vi "GeoData.vi"() -> ()   [LabVIEW 2017] (continued)
KS\tCloud County\tH1\n67466\t20029\tMiltonvale\tKS\tCloud County\tH1\n67417\t20029\tAurora\tKS\tCloud County\tH1\n66930\t20029\tAgenda\tKS\tCloud County\tH1\n67420\t20029\tBeloit\tKS\tCloud County\tH1\n66948\t20029\tJamestown\tKS\tCloud County\tH1\n67436\t20029\tDelphos\tKS\tCloud County\tH1\n67445\t20029\tGlasco\tKS\tCloud County\tH1\n66938\t20029\tClyde\tKS\tCloud County\tH1\n66783\t20031\tYates center\tKS\tCoffey County\tH1\n66868\t20031\tReading\tKS\tCoffey County\tH1\n66093\t20031\tWestphalia\tKS\tCoffey County\tH1\n66854\t20031\tHartford\tKS\tCoffey County\tH1\n66856\t20031\tLebo\tKS\tCoffey County\tH1\n66839\t20031\tBurlington\tKS\tCoffey County\tH1\n66864\t20031\tNeosho rapids\tKS\tCoffey County\tH1\n66857\t20031\tLe roy\tKS\tCoffey County\tH1\n66095\t20031\tWilliamsburg\tKS\tCoffey County\tH1\n66852\t20031\tGridley\tKS\tCoffey County\tH1\n66758\t20031\tNeosho falls\tKS\tCoffey County\tH1\n66871\t20031\tWaverly\tKS\tCoffey County\tH1\n67029\t20033\tColdwater\tKS\tComanche County\tH1\n67155\t20033\tWilmore\tKS\tComanche County\tH1\n67127\t20033\tProtection\tKS\tComanche County\tH1\n67005\t20035\tArkansas city\tKS\tCowley County\tH1\n67119\t20035\tOxford\tKS\tCowley County\tH1\n67110\t20035\tMulvane\tKS\tCowley County\tH1\n67072\t20035\tLatham\tKS\tCowley County\tH1\n67102\t20035\tMaple city\tKS\tCowley County\tH1\n67008\t20035\tAtlanta\tKS\tCowley County\tH1\n67051\t20035\tGeuda springs\tKS\tCowley County\tH1\n67023\t20035\tCambridge\tKS\tCowley County\tH1\n67039\t20035\tDouglass\tKS\tCowley County\tH1\n67024\t20035\tCedar vale\tKS\tCowley County\tH1\n67131\t20035\tRock\tKS\tCowley County\tH1\n67038\t20035\tDexter\tKS\tCowley County\tH1\n67146\t20035\tUdall\tKS\tCowley County\tH1\n67156\t20035\tWinfield\tKS\tCowley County\tH1\n67019\t20035\tBurden\tKS\tCowley County\tH1\n66712\t20037\tArma\tKS\tCrawford County\tH1\n66746\t20037\tHepler\tKS\tCrawford County\tH1\n66701\t20037\tFort scott\tKS\tCrawford County\tH1\n66743\t20037\tGirard\tKS\tCrawford County\tH1\n66711\t20037\tArcadia\tKS\tCrawford County\tH1\n66724\t20037\tCherokee\tKS\tCrawford County\tH1\n66734\t20037\tFarlington\tKS\tCrawford County\tH1\n66760\t20037\tOpolis\tKS\tCrawford County\tH1\n66763\t20037\tFrontenac\tKS\tCrawford County\tH1\n66756\t20037\tMulberry\tKS\tCrawford County\tH1\n66762\t20037\tPittsburg\tKS\tCrawford County\tH1\n66735\t20037\tFranklin\tKS\tCrawford County\tH1\n66781\t20037\tWeir\tKS\tCrawford County\tH1\n66753\t20037\tMc cune\tKS\tCrawford County\tH1\n66780\t20037\tWalnut\tKS\tCrawford County\tH1\n67749\t20039\tOberlin\tKS\tDecatur County\tH1\n67757\t20039\tSelden\tKS\tDecatur County\tH1\n67643\t20039\tJennings\tKS\tDecatur County\tH1\n67653\t20039\tNorcatur\tKS\tDecatur County\tH1\n67635\t20039\tDresden\tKS\tDecatur County\tH1\n66441\t20041\tJunction city\tKS\tDickinson County\tH1\n67410\t20041\tAbilene\tKS\tDickinson County\tH1\n67448\t20041\tGypsum\tKS\tDickinson County\tH1\n67451\t20041\tHope\tKS\tDickinson County\tH1\n67480\t20041\tSolomon\tKS\tDickinson County\tH1\n67475\t20041\tRamona\tKS\tDickinson County\tH1\n67449\t20041\tHerington\tKS\tDickinson County\tH1\n67441\t20041\tEnterprise\tKS\tDickinson County\tH1\n67492\t20041\tWoodbine\tKS\tDickinson County\tH1\n67431\t20041\tChapman\tKS\tDickinson County\tH1\n67487\t20041\tWakefield\tKS\tDickinson County\tH1\n67482\t20041\tTalmage\tKS\tDickinson County\tH1\n66094\t20043\tWhite cloud\tKS\tDoniphan County\tH1\n66087\t20043\tTroy\tKS\tDoniphan County\tH1\n66017\t20043\tDenton\tKS\tDoniphan County\tH1\n66090\t20043\tWathena\tKS\tDoniphan County\tH1\n66024\t20043\tElwood\tKS\tDoniphan County\tH1\n66041\t20043\tLancaster\tKS\tDoniphan County\tH1\n66008\t20043\tBendena\tKS\tDoniphan County\tH1\n66035\t20043\tHighland\tKS\tDoniphan County\tH1\n66002\t20043\tAtchison\tKS\tDoniphan County\tH1\n66532\t20043\tRobinson\tKS\tDoniphan County\tH1\n66049\t20045\tLawrence\tKS\tDouglas County\tH1\n66025\t20045\tEudora\tKS\tDouglas County\tH1\n66050\t20045\tLecompton\tKS\tDouglas County\tH1\n66046\t20045\tLawrence\tKS\tDouglas County\tH1\n66092\t20045\tWellsville\tKS\tDouglas County\tH1\n66021\t20045\tEdgerton\tKS\tDouglas County\tH1\n66409\t20045\tBerryton\tKS\tDouglas County\tH1\n66524\t20045\tOverbrook\tKS\tDouglas County\tH1\n66047\t20045\tLawrence\tKS\tDouglas County\tH1\n66542\t20045\tTecumseh\tKS\tDouglas County\tH1\n66045\t20045\tLawrence\tKS\tDouglas County\tH1\n66006\t20045\tBaldwin city\tKS\tDouglas County\tH1\n66044\t20045\tLawrence\tKS\tDouglas County\tH1\n67054\t20047\tGreensburg\tKS\tEdwards County\tH1\n67563\t20047\tOfferle\tKS\tEdwards County\tH1\n67519\t20047\tBelpre\tKS\tEdwards County\tH1\n67059\t20047\tHaviland\tKS\tEdwards County\tH1\n67547\t20047\tKinsley\tKS\tEdwards County\tH1\n67557\t20047\tMacksville\tKS\tEdwards County\tH1\n67552\t20047\tLewis\tKS\tEdwards County\tH1\n67344\t20049\tElk city\tKS\tElk County\tH1\n67353\t20049\tMoline\tKS\tElk County\tH1\n67345\t20049\tElk falls\tKS\tElk County\tH1\n67346\t20049\tGrenola\tKS\tElk County\tH1\n67122\t20049\tPiedmont\tKS\tElk County\tH1\n67137\t20049\tSevery\tKS\tElk County\tH1\n67047\t20049\tFall river\tKS\tElk County\tH1\n67349\t20049\tHoward\tKS\tElk County\tH1\n67352\t20049\tLongton\tKS\tElk County\tH1\n67640\t20051\tGorham\tKS\tEllis County\tH1\n67659\t20051\tPenokee\tKS\tEllis County\tH1\n67660\t20051\tPfeifer\tKS\tEllis County\tH1\n67651\t20051\tNatoma\tKS\tEllis County\tH1\n67663\t20051\tPlainville\tKS\tEllis County\tH1\n67627\t20051\tCatharine\tKS\tEllis County\tH1\n67671\t20051\tVictoria\tKS\tEllis County\tH1\n67667\t20051\tSchoenchen\tKS\tEllis County\tH1\n67601\t20051\tHays\tKS\tEllis County\tH1\n67674\t20051\tWalker\tKS\tEllis County\tH1\n67637\t20051\tEllis\tKS\tEllis County\tH1\n67556\t20051\tMc cracken\tKS\tEllis County\tH1\n67520\t20051\tBison\tKS\tEllis County\tH1\n67423\t20053\tBeverly\tKS\tEllsworth County\tH1\n67459\t20053\tLorraine\tKS\tEllsworth County\tH1\n67450\t20053\tHolyrood\tKS\tEllsworth County\tH1\n67439\t20053\tEllsworth\tKS\tEllsworth County\tH1\n67425\t20053\tBrookville\tKS\tEllsworth County\tH1\n67444\t20053\tGeneseo\tKS\tEllsworth County\tH1\n67490\t20053\tWilson\tKS\tEllsworth County\tH1\n67427\t20053\tBushton\tKS\tEllsworth County\tH1\n67464\t20053\tMarquette\tKS\tEllsworth County\tH1\n67454\t20053\tKanopolis\tKS\tEllsworth County\tH1\n67851\t20055\tHolcomb\tKS\tFinney County\tH1\n67839\t20055\tDighton\tKS\tFinney County\tH1\n67838\t20055\tDeerfield\tKS\tFinney County\tH1\n67871\t20055\tScott city\tKS\tFinney County\tH1\n67853\t20055\tIngalls\tKS\tFinney County\tH1\n67868\t20055\tPierceville\tKS\tFinney County\tH1\n67846\t20055\tGarden city\tKS\tFinney County\tH1\n67835\t20055\tCimarron\tKS\tFinney County\tH1\n67834\t20057\tBucklin\tKS\tFord County\tH1\n67563\t20057\tOfferle\tKS\tFord County\tH1\n67842\t20057\tFord\tKS\tFord County\tH1\n67844\t20057\tFowler\tKS\tFord County\tH1\n67865\t20057\tMinneola\tKS\tFord County\tH1\n67801\t20057\tDodge city\tKS\tFord County\tH1\n67882\t20057\tWright\tKS\tFord County\tH1\n67876\t20057\tSpearville\tKS\tFord County\tH1\n67841\t20057\tEnsign\tKS\tFord County\tH1\n67835\t20057\tCimarron\tKS\tFord County\tH1\n66033\t20059\tGreeley\tKS\tFranklin County\tH1\n66079\t20059\tRantoul\tKS\tFranklin County\tH1\n66076\t20059\tPomona\tKS\tFranklin County\tH1\n66078\t20059\tPrinceton\tKS\tFranklin County\tH1\n66092\t20059\tWellsville\tKS\tFranklin County\tH1\n66080\t20059\tRichmond\tKS\tFranklin County\tH1\n66524\t20059\tOverbrook\tKS\tFranklin County\tH1\n66067\t20059\tOttawa\tKS\tFranklin County\tH1\n66095\t20059\tWilliamsburg\tKS\tFranklin County\tH1\n66042\t20059\tLane\tKS\tFranklin County\tH1\n66528\t20059\tQuenemo\tKS\tFranklin County\tH1\n66006\t20059\tBaldwin city\tKS\tFranklin County\tH1\n66064\t20059\tOsawatomie\tKS\tFranklin County\tH1\n66441\t20061\tJunction city\tKS\tGeary County\tH1\n66442\t20061\tFort riley\tKS\tGeary County\tH1\n66401\t20061\tAlma\tKS\tGeary County\tH1\n66834\t20061\tAlta vista\tKS\tGeary County\tH1\n66502\t20061\tManhattan\tKS\tGeary County\tH1\n66849\t20061\tDwight\tKS\tGeary County\tH1\n66872\t20061\tWhite city\tKS\tGeary County\tH1\n67431\t20061\tChapman\tKS\tGeary County\tH1\n66514\t20061\tMilford\tKS\tGeary County\tH1\n67487\t20061\tWakefield\tKS\tGeary County\tH1\n67748\t20063\tOakley\tKS\tGove County\tH1\n67752\t20063\tQuinter\tKS\tGove County\tH1\n67751\t20063\tPark\tKS\tGove County\tH1\n67738\t20063\tGrinnell\tKS\tGove County\tH1\n67737\t20063\tGrainfield\tKS\tGove County\tH1\n67736\t20063\tGove\tKS\tGove County\tH1\n67625\t20065\tBogue\tKS\tGraham County\tH1\n67656\t20065\tOgallah\tKS\tGraham County\tH1\n67650\t20065\tMorland\tKS\tGraham County\tH1\n67659\t20065\tPenokee\tKS\tGraham County\tH1\n67642\t20065\tHill city\tKS\tGraham County\tH1\n67740\t20065\tHoxie\tKS\tGraham County\tH1\n67632\t20065\tDamar\tKS\tGraham County\tH1\n67657\t20065\tPalco\tKS\tGraham County\tH1\n67672\t20065\tWakeeney\tKS\tGraham County\tH1\n67855\t20067\tJohnson\tKS\tGrant County\tH1\n67880\t20067\tUlysses\tKS\tGrant County\tH1\n67870\t20067\tSatanta\tKS\tGrant County\tH1\n67860\t20067\tLakin\tKS\tGrant County\tH1\n67844\t20069\tFowler\tKS\tGray County\tH1\n67853\t20069\tIngalls\tKS\tGray County\tH1\n67801\t20069\tDodge city\tKS\tGray County\tH1\n67867\t20069\tMontezuma\tKS\tGray County\tH1\n67843\t20069\tFort dodge\tKS\tGray County\tH1\n67841\t20069\tEnsign\tKS\tGray County\tH1\n67846\t20069\tGarden city\tKS\tGray County\tH1\n67837\t20069\tCopeland\tKS\tGray County\tH1\n67835\t20069\tCimarron\tKS\tGray County\tH1\n67879\t20071\tTribune\tKS\tGreeley County\tH1\n67762\t20071\tWeskan\tKS\tGreeley County\tH1\n66870\t20073\tVirgil\tKS\tGreenwood County\tH1\n66853\t20073\tHamilton\tKS\tGreenwood County\tH1\n67045\t20073\tEureka\tKS\tGreenwood County\tH1\n66860\t20073\tMadison\tKS\tGreenwood County\tH1\n67122\t20073\tPiedmont\tKS\tGreenwood County\tH1\n66852\t20073\tGridley\tKS\tGreenwood County\tH1\n67137\t20073\tSevery\tKS\tGreenwood County\tH1\n67047\t20073\tFall river\tKS\tGreenwood County\tH1\n66777\t20073\tToronto\tKS\tGreenwood County\tH1\n66855\t20073\tLamont\tKS\tGreenwood County\tH1\n66863\t20073\tNeal\tKS\tGreenwood County\tH1\n67857\t20075\tKendall\tKS\tHamilton County\tH1\n67878\t20075\tSyracuse\tKS\tHamilton County\tH1\n67836\t20075\tCoolidge\tKS\tHamilton County\tH1\n67009\t20077\tAttica\tKS\tHarper County\tH1\n67159\t20077\tZenda\tKS\tHarper County\tH1\n67058\t20077\tHarper\tKS\tHarper County\tH1\n67138\t20077\tSharon\tKS\tHarper County\tH1\n67049\t20077\tFreeport\tKS\tHarper County\tH1\n67003\t20077\tAnthony\tKS\tHarper County\tH1\n67061\t20077\tHazelton\tKS\tHarper County\tH1\n67036\t20077\tDanville\tKS\tHarper County\tH1\n67004\t20077\tArgonia\tKS\tHarper County\tH1\n67018\t20077\tBluff city\tKS\tHarper County\tH1\n67150\t20077\tWaldron\tKS\tHarper County\tH1\n67117\t20079\tNorth newton\tKS\tHarvey County\tH1\n67522\t20079\tBuhler\tKS\tHarvey County\tH1\n67020\t20079\tBurrton\tKS\tHarvey County\tH1\n66866\t20079\tPeabody\tKS\tHarvey County\tH1\n67546\t20079\tInman\tKS\tHarvey County\tH1\n67135\t20079\tSedgwick\tKS\tHarvey County\tH1\n67147\t20079\tValley center\tKS\tHarvey County\tH1\n67062\t20079\tHesston\tKS\tHarvey County\tH1\n67114\t20079\tNewton\tKS\tHarvey County\tH1\n67151\t20079\tWalton\tKS\tHarvey County\tH1\n67154\t20079\tWhitewater\tKS\tHarvey County\tH1\n67107\t20079\tMoundridge\tKS\tHarvey County\tH1\n67056\t20079\tHalstead\tKS\tHarvey County\tH1\n67880\t20081\tUlysses\tKS\tHaskell County\tH1\n67870\t20081\tSatanta\tKS\tHaskell County\tH1\n67877\t20081\tSublette\tKS\tHaskell County\tH1\n67837\t20081\tCopeland\tKS\tHaskell County\tH1\n67952\t20081\tMoscow\tKS\tHaskell County\tH1\n67854\t20083\tJetmore\tKS\tHodgeman County\tH1\n67563\t20083\tOfferle\tKS\tHodgeman County\tH1\n67801\t20083\tDodge city\tKS\tHodgeman County\tH1\n67849\t20083\tHanston\tKS\tHodgeman County\tH1\n67876\t20083\tSpearville\tKS\tHodgeman County\tH1\n67547\t20083\tKinsley\tKS\tHodgeman County\tH1\n67523\t20083\tBurdett\tKS\tHodgeman County\tH1\n67835\t20083\tCimarron\tKS\tHodgeman County\tH1\n66058\t20085\tMuscotah\tKS\tJackson County\tH1\n66539\t20085\tSilver lake\tKS\tJackson County\tH1\n66617\t20085\tTopeka\tKS\tJackson County\tH1\n66512\t20085\tMeriden\tKS\tJackson County\tH1\n66536\t20085\tSaint marys\tKS\tJackson County\tH1\n66552\t20085\tWhiting\tKS\tJackson County\tH1\n66416\t20085\tCircleville\tKS\tJackson County\tH1\n66422\t20085\tEmmett\tKS\tJackson County\tH1\n66509\t20085\tMayetta\tKS\tJackson County\tH1\n66516\t20085\tNetawaka\tKS\tJackson County\tH1\n66432\t20085\tHavensville\tKS\tJackson County\tH1\n66540\t20085\tSoldier\tKS\tJackson County\tH1\n66436\t20085\tHolton\tKS\tJackson County\tH1\n66418\t20085\tDelia\tKS\tJackson County\tH1\n66439\t20085\tHorton\tKS\tJackson County\tH1\n66533\t20085\tRossville\tKS\tJackson County\tH1\n66419\t20085\tDenison\tKS\tJackson County\tH1\n66440\t20085\tHoyt\tKS\tJackson County\tH1\n66618\t20085\tTopeka\tKS\tJackson County\tH1\n66550\t20085\tWetmore\tKS\tJackson County\tH1\n66086\t20087\tTonganoxie\tKS\tJefferson County\tH1\n66073\t20087\tPerry\tKS\tJefferson County\tH1\n66617\t20087\tTopeka\tKS\tJefferson County\tH1\n66512\t20087\tMeriden\tKS\tJefferson County\tH1\n66429\t20087\tGrantville\tKS\tJefferson County\tH1\n66088\t20087\tValley falls\tKS\tJefferson County\tH1\n66054\t20087\tMc louth\tKS\tJefferson County\tH1\n66097\t20087\tWinchester\tKS\tJefferson County\tH1\n66002\t20087\tAtchison\tKS\tJefferson County\tH1\n66066\t20087\tOskaloosa\tKS\tJefferson County\tH1\n66070\t20087\tOzawkie\tKS\tJefferson County\tH1\n66436\t20087\tHolton\tKS\tJefferson County\tH1\n66419\t20087\tDenison\tKS\tJefferson County\tH1\n66044\t20087\tLawrence\tKS\tJefferson County\tH1\n66060\t20087\tNortonville\tKS\tJefferson County\tH1\n66939\t20089\tCourtland\tKS\tJewell County\tH1\n66956\t20089\tMankato\tKS\tJewell County\tH1\n66941\t20089\tEsbon\tKS\tJewell County\tH1\n66970\t20089\tWebber\tKS\tJewell County\tH1\n67420\t20089\tBeloit\tKS\tJewell County\tH1\n66949\t20089\tJewell\tKS\tJewell County\tH1\n66948\t20089\tJamestown\tKS\tJewell County\tH1\n66963\t20089\tRandall\tKS\tJewell County\tH1\n66936\t20089\tBurr oak\tKS\tJewell County\tH1\n67430\t20089\tCawker city\tKS\tJewell County\tH1\n66942\t20089\tFormoso\tKS\tJewell County\tH1\n66083\t20091\tSpring hill\tKS\tJohnson County\tH1\n66025\t20091\tEudora\tKS\tJohnson County\tH1\n66031\t20091\tNew century\tKS\tJohnson County\tH1\n66250\t20091\tLenexa\tKS\tJohnson County\tH1\n66018\t20091\tDe soto\tKS\tJohnson County\tH1\n66013\t20091\tBucyrus\tKS\tJohnson County\tH1\n66204\t20091\tOverland park\tKS\tJohnson County\tH1\n66210\t20091\tOverland park\tKS\tJohnson County\tH1\n66085\t20091\tStilwell\tKS\tJohnson County\tH1\n66283\t20091\tOverland park\tKS\tJohnson County\tH1\n66208\t20091\tPrairie village\tKS\tJohnson County\tH1\n66211\t20091\tLeawood\tKS\tJohnson County\tH1\n66213\t20091\tOverland park\tKS\tJohnson County\tH1\n66106\t20091\tKansas city\tKS\tJohnson County\tH1\n66205\t20091\tMission\tKS\tJohnson County\tH1\n66216\t20091\tShawnee\tKS\tJohnson County\tH1\n66218\t20091\tShawnee\tKS\tJohnson County\tH1\n66286\t20091\tShawnee\tKS\tJohnson County\tH1\n66051\t20091\tOlathe\tKS\tJohnson County\tH1\n66061\t20091\tOlathe\tKS\tJohnson County\tH1\n66021\t20091\tEdgerton\tKS\tJohnson County\tH1\n66206\t20091\tLeawood\tKS\tJohnson County\tH1\n66217\t20091\tShawnee\tKS\tJohnson County\tH1\n66214\t20091\tOverland park\tKS\tJohnson County\tH1\n66221\t20091\tOverland park\tKS\tJohnson County\tH1\n66223\t20091\tOverland park\tKS\tJohnson County\tH1\n66227\t20091\tLenexa\tKS\tJohnson County\tH1\n66282\t20091\tOverland park\tKS\tJohnson County\tH1\n66212\t20091\tOverland park\tKS\tJohnson County\tH1\n66219\t20091\tLenexa\tKS\tJohnson County\tH1\n66276\t20091\tLenexa\tKS\tJohnson County\tH1\n66030\t20091\tGardner\tKS\tJohnson County\tH1\n66203\t20091\tShawnee\tKS\tJohnson County\tH1\n66285\t20091\tLenexa\tKS\tJohnson County\tH1\n66063\t20091\tOlathe\tKS\tJohnson County\tH1\n66251\t20091\tOverland park\tKS\tJohnson County\tH1\n66209\t20091\tLeawood\tKS\tJohnson County\tH1\n66215\t20091\tLenexa\tKS\tJohnson County\tH1\n66207\t20091\tOverland park\tKS\tJohnson County\tH1\n66220\t20091\tLenexa\tKS\tJohnson County\tH1\n66225\t20091\tOverland park\tKS\tJohnson County\tH1\n66062\t20091\tOlathe\tKS\tJohnson County\tH1\n66202\t20091\tMission\tKS\tJohnson County\tH1\n66224\t20091\tOverland park\tKS\tJohnson County\tH1\n66226\t20091\tShawnee\tKS\tJohnson County\tH1\n66201\t20091\tMission\tKS\tJohnson County\tH1\n67838\t20093\tDeerfield\tKS\tKearny County\tH1\n67880\t20093\tUlysses\tKS\tKearny County\tH1\n67860\t20093\tLakin\tKS\tKearny County\tH1\n67025\t20095\tCheney\tKS\tKingman County\tH1\n67035\t20095\tCunningham\tKS\tKingman County\tH1\n67112\t20095\tNashville\tKS\tKingman County\tH1\n67159\t20095\tZenda\tKS\tKingman County\tH1\n67058\t20095\tHarper\tKS\tKingman County\tH1\n67068\t20095\tKingman\tKS\tKingman County\tH1\n67111\t20095\tMurdock\tKS\tKingman County\tH1\n67142\t20095\tSpivey\tKS\tKingman County\tH1\n67004\t20095\tArgonia\tKS\tKingman County\tH1\n67570\t20095\tPretty prairie\tKS\tKingman County\tH1\n67118\t20095\tNorwich\tKS\tKingman County\tH1\n67054\t20097\tGreensburg\tKS\tKiowa County\tH1\n67109\t20097\tMullinville\tKS\tKiowa County\tH1\n67834\t20097\tBucklin\tKS\tKiowa County\tH1\n67028\t20097\tCoats\tKS\tKiowa County\tH1\n67059\t20097\tHaviland\tKS\tKiowa County\tH1\n67336\t20099\tChetopa\tKS\tLabette County\tH1\n67332\t20099\tBartlett\tKS\tLabette County\tH1\n67341\t20099\tDennis\tKS\tLabette County\tH1\n67337\t20099\tCoffeyville\tKS\tLabette County\tH1\n66776\t20099\tThayer\tKS\tLabette County\tH1\n67351\t20099\tLiberty\tKS\tLabette County\tH1\n67356\t20099\tOswego\tKS\tLabette County\tH1\n67357\t20099\tParsons\tKS\tLabette County\tH1\n67342\t20099\tEdna\tKS\tLabette County\tH1\n67330\t20099\tAltamont\tKS\tLabette County\tH1\n67335\t20099\tCherryvale\tKS\tLabette County\tH1\n66753\t20099\tMc cune\tKS\tLabette County\tH1\n67354\t20099\tMound valley\tKS\tLabette County\tH1\n67839\t20101\tDighton\tKS\tLane County\tH1\n67850\t20101\tHealy\tKS\tLane County\tH1\n67846\t20101\tGarden city\tKS\tLane County\tH1\n66086\t20103\tTonganoxie\tKS\tLeavenworth County\tH1\n66020\t20103\tEaston\tKS\tLeavenworth County\tH1\n66048\t20103\tLeavenworth\tKS\tLeavenworth County\tH1\n66007\t20103\tBasehor\tKS\tLeavenworth County\tH1\n66027\t20103\tFort leavenworth\tKS\tLeavenworth County\tH1\n66043\t20103\tLansing\tKS\tLeavenworth County\tH1\n66054\t20103\tMc louth\tKS\tLeavenworth County\tH1\n66097\t20103\tWinchester\tKS\tLeavenworth County\tH1\n66002\t20103\tAtchison\tKS\tLeavenworth County\tH1\n66012\t20103\tBonner springs\tKS\tLeavenworth County\tH1\n66052\t20103\tLinwood\tKS\tLeavenworth County\tH1\n66109\t20103\tKansas city\tKS\tLeavenworth County\tH1\n66044\t20103\tLawrence\tKS\tLeavenworth County\tH1\n67455\t20105\tLincoln\tKS\tLincoln County\tH1\n67423\t20105\tBeverly\tKS\tLincoln County\tH1\n67467\t20105\tMinneapolis\tKS\tLincoln County\tH1\n67490\t20105\tWilson\tKS\tLincoln County\tH1\n67648\t20105\tLucas\tKS\tLincoln County\tH1\n67452\t20105\tHunter\tKS\tLincoln County\tH1\n67481\t20105\tSylvan grove\tKS\tLincoln County\tH1\n67484\t20105\tTescott\tKS\tLincoln County\tH1\n67418\t20105\tBarnard\tKS\tLincoln County\tH1\n66014\t20107\tCenterville\tKS\tLinn County\tH1\n66075\t20107\tPleasanton\tKS\tLinn County\tH1\n66033\t20107\tGreeley\tKS\tLinn County\tH1\n66738\t20107\tFulton\tKS\tLinn County\tH1\n66026\t20107\tFontana\tKS\tLinn County\tH1\n66767\t20107\tPrescott\tKS\tLinn County\tH1\n66754\t20107\tMapleton\tKS\tLinn County\tH1\n66010\t20107\tBlue mound\tKS\tLinn County\tH1\n66042\t20107\tLane\tKS\tLinn County\tH1\n66064\t20107\tOsawatomie\tKS\tLinn County\tH1\n66056\t20107\tMound city\tKS\tLinn County\tH1\n66040\t20107\tLa cygne\tKS\tLinn County\tH1\n66072\t20107\tParker\tKS\tLinn County\tH1\n67748\t20109\tOakley\tKS\tLogan County\tH1\n67861\t20109\tLeoti\tKS\tLogan County\tH1\n67732\t20109\tBrewster\tKS\tLogan County\tH1\n67871\t20109\tScott city\tKS\tLogan County\tH1\n67764\t20109\tWinona\tKS\tLogan County\tH1\n67747\t20109\tMonument\tKS\tLogan County\tH1\n67761\t20109\tWallace\tKS\tLogan County\tH1\n66868\t20111\tReading\tKS\tLyon County\tH1\n66830\t20111\tAdmire\tKS\tLyon County\tH1\n66854\t20111\tHartford\tKS\tLyon County\tH1\n66860\t20111\tMadison\tKS\tLyon County\tH1\n66864\t20111\tNeosho rapids\tKS\tLyon County\tH1\n66846\t20111\tCouncil grove\tKS\tLyon County\tH1\n66523\t20111\tOsage city\tKS\tLyon County\tH1\n66833\t20111\tAllen\tKS\tLyon County\tH1\n66801\t20111\tEmporia\tKS\tLyon County\tH1\n66835\t20111\tAmericus\tKS\tLyon County\tH1\n66865\t20111\tOlpe\tKS\tLyon County\tH1\n67448\t20113\tGypsum\tKS\tMcPherson County\tH1\n67546\t20113\tInman\tKS\tMcPherson County\tH1\n67416\t20113\tAssaria\tKS\tMcPherson County\tH1\n67062\t20113\tHesston\tKS\tMcPherson County\tH1\n67443\t20113\tGalva\tKS\tMcPherson County\tH1\n67460\t20113\tMcpherson\tKS\tMcPherson County\tH1\n67456\t20113\tLindsborg\tKS\tMcPherson County\tH1\n67491\t20113\tWindom\tKS\tMcPherson County\tH1\n67464\t20113\tMarquette\tKS\tMcPherson County\tH1\n67107\t20113\tMoundridge\tKS\tMcPherson County\tH1\n67428\t20113\tCanton\tKS\tMcPherson County\tH1\n67476\t20113\tRoxbury\tKS\tMcPherson County\tH1\n66869\t20115\tStrong city\tKS\tMarion County\tH1\n67483\t20115\tTampa\tKS\tMarion County\tH1\n66866\t20115\tPeabody\tKS\tMarion County\tH1\n67063\t20115\tHillsboro\tKS\tMarion County\tH1\n67451\t20115\tHope\tKS\tMarion County\tH1\n67053\t20115\tGoessel\tKS\tMarion County\tH1\n67438\t20115\tDurham\tKS\tMarion County\tH1\n67475\t20115\tRamona\tKS\tMarion County\tH1\n66861\t20115\tMarion\tKS\tMarion County\tH1\n67073\t20115\tLehigh\tKS\tMarion County\tH1\n66838\t20115\tBurdick\tKS\tMarion County\tH1\n67114\t20115\tNewton\tKS\tMarion County\tH1\n66840\t20115\tBurns\tKS\tMarion County\tH1\n67151\t20115\tWalton\tKS\tMarion County\tH1\n66843\t20115\tCedar point\tKS\tMarion County\tH1\n66858\t20115\tLincolnville\tKS\tMarion County\tH1\n66859\t20115\tLost springs\tKS\tMarion County\tH1\n66851\t20115\tFlorence\tKS\tMarion County\tH1\n67428\t20115\tCanton\tKS\tMarion County\tH1\n66406\t20117\tBeattie\tKS\tMarshall County\tH1\n66508\t20117\tMarysville\tKS\tMarshall County\tH1\n66548\t20117\tWaterville\tKS\tMarshall County\tH1\n66521\t20117\tOnaga\tKS\tMarshall County\tH1\n66541\t20117\tSummerfield\tKS\tMarshall County\tH1\n66945\t20117\tHanover\tKS\tMarshall County\tH1\n66518\t20117\tOketo\tKS\tMarshall County\tH1\n66412\t20117\tBremen\tKS\tMarshall County\tH1\n66411\t20117\tBlue rapids\tKS\tMarshall County\tH1\n66427\t20117\tFrankfort\tKS\tMarshall County\tH1\n66544\t20117\tVermillion\tKS\tMarshall County\tH1\n66403\t20117\tAxtell\tKS\tMarshall County\tH1\n66404\t20117\tBaileyville\tKS\tMarshall County\tH1\n66438\t20117\tHome\tKS\tMarshall County\tH1\n67869\t20119\tPlains\tKS\tMeade County\tH1\n67844\t20119\tFowler\tKS\tMeade County\tH1\n67867\t20119\tMontezuma\tKS\tMeade County\tH1\n67841\t20119\tEnsign\tKS\tMeade County\tH1\n67864\t20119\tMeade\tKS\tMeade County\tH1\n66083\t20121\tSpring hill\tKS\tMiami County\tH1\n66079\t20121\tRantoul\tKS\tMiami County\tH1\n66013\t20121\tBucyrus\tKS\tMiami County\tH1\n66026\t20121\tFontana\tKS\tMiami County\tH1\n66036\t20121\tHillsdale\tKS\tMiami County\tH1\n66092\t20121\tWellsville\tKS\tMiami County\tH1\n66021\t20121\tEdgerton\tKS\tMiami County\tH1\n66053\t20121\tLouisburg\tKS\tMiami County\tH1\n66071\t20121\tPaola\tKS\tMiami County\tH1\n66030\t20121\tGardner\tKS\tMiami County\tH1\n66042\t20121\tLane\tKS\tMiami County\tH1\n66064\t20121\tOsawatomie\tKS\tMiami County\tH1\n66040\t20121\tLa cygne\tKS\tMiami County\tH1\n66072\t20121\tParker\tKS\tMiami County\tH1\n67485\t20123\tTipton\tKS\tMitchell County\tH1\n67420\t20123\tBeloit\tKS\tMitchell County\tH1\n67446\t20123\tGlen elder\tKS\tMitchell County\tH1\n67430\t20123\tCawker city\tKS\tMitchell County\tH1\n67452\t20123\tHunter\tKS\tMitchell County\tH1\n67478\t20123\tSimpson\tKS\tMitchell County\tH1\n67418\t20123\tBarnard\tKS\tMitchell County\tH1\n67344\t20125\tElk city\tKS\tMontgomery County\tH1\n66736\t20125\tFredonia\tKS\tMontgomery County\tH1\n67337\t20125\tCoffeyville\tKS\tMontgomery County\tH1\n67347\t20125\tHavana\tKS\tMontgomery County\tH1\n66757\t20125\tNeodesha\tKS\tMontgomery County\tH1\n67301\t20125\tIndependence\tKS\tMontgomery County\tH1\n67351\t20125\tLiberty\tKS\tMontgomery County\tH1\n67340\t20125\tDearing\tKS\tMontgomery County\tH1\n67364\t20125\tTyro\tKS\tMontgomery County\tH1\n67335\t20125\tCherryvale\tKS\tMontgomery County\tH1\n67363\t20125\tSycamore\tKS\tMontgomery County\tH1\n67333\t20125\tCaney\tKS\tMontgomery County\tH1\n66873\t20127\tWilsey\tKS\tMorris County\tH1\n66834\t20127\tAlta vista\tKS\tMorris County\tH1\n67449\t20127\tHerington\tKS\tMorris County\tH1\n66838\t20127\tBurdick\tKS\tMorris County\tH1\n66846\t20127\tCouncil grove\tKS\tMorris County\tH1\n66849\t20127\tDwight\tKS\tMorris County\tH1\n66872\t20127\tWhite city\tKS\tMorris County\tH1\n66859\t20127\tLost springs\tKS\tMorris County\tH1\n67954\t20129\tRolla\tKS\tMorton County\tH1\n67953\t20129\tRichfield\tKS\tMorton County\tH1\n67950\t20129\tElkhart\tKS\tMorton County\tH1\n66521\t20131\tOnaga\tKS\tNemaha County\tH1\n66408\t20131\tBern\tKS\tNemaha County\tH1\n66428\t20131\tGoff\tKS\tNemaha County\tH1\n66534\t20131\tSabetha\tKS\tNemaha County\tH1\n66522\t20131\tOneida\tKS\tNemaha County\tH1\n66416\t20131\tCircleville\tKS\tNemaha County\tH1\n66538\t20131\tSeneca\tKS\tNemaha County\tH1\n66432\t20131\tHavensville\tKS\tNemaha County\tH1\n66540\t20131\tSoldier\tKS\tNemaha County\tH1\n66417\t20131\tCorning\tKS\tNemaha County\tH1\n66415\t20131\tCentralia\tKS\tNemaha County\tH1\n66544\t20131\tVermillion\tKS\tNemaha County\tH1\n66403\t20131\tAxtell\tKS\tNemaha County\tH1\n66404\t20131\tBaileyville\tKS\tNemaha County\tH1\n66550\t20131\tWetmore\tKS\tNemaha County\tH1\n67341\t20133\tDennis\tKS\tNeosho County\tH1\n66775\t20133\tStark\tKS\tNeosho County\tH1\n66748\t20133\tHumboldt\tKS\tNeosho County\tH1\n66740\t20133\tGalesburg\tKS\tNeosho County\tH1\n66776\t20133\tThayer\tKS\tNeosho County\tH1\n66771\t20133\tSaint paul\tKS\tNeosho County\tH1\n67357\t20133\tParsons\tKS\tNeosho County\tH1\n66733\t20133\tErie\tKS\tNeosho County\tH1\n66753\t20133\tMc cune\tKS\tNeosho County\tH1\n66720\t20133\tChanute\tKS\tNeosho County\tH1\n66780\t20133\tWalnut\tKS\tNeosho County\tH1\n66772\t20133\tSavonburg\tKS\tNeosho County\tH1\n67518\t20135\tBeeler\tKS\tNess County\tH1\n67584\t20135\tUtica\tKS\tNess County\tH1\n67572\t20135\tRansom\tKS\tNess County\tH1\n67515\t20135\tArnold\tKS\tNess County\tH1\n67516\t20135\tBazine\tKS\tNess County\tH1\n67560\t20135\tNess city\tKS\tNess County\tH1\n67521\t20135\tBrownell\tKS\tNess County\tH1\n67629\t20137\tClayton\tKS\tNorton County\tH1\n67653\t20137\tNorcatur\tKS\tNorton County\tH1\n67645\t20137\tLenora\tKS\tNorton County\tH1\n67622\t20137\tAlmena\tKS\tNorton County\tH1\n67654\t20137\tNorton\tKS\tNorton County\tH1\n66414\t20139\tCarbondale\tKS\tOsage County\tH1\n66868\t20139\tReading\tKS\tOsage County\tH1\n66537\t20139\tScranton\tKS\tOsage County\tH1\n66413\t20139\tBurlingame\tKS\tOsage County\tH1\n66409\t20139\tBerryton\tKS\tOsage County\tH1\n66524\t20139\tOverbrook\tKS\tOsage County\tH1\n66856\t20139\tLebo\tKS\tOsage County\tH1\n66095\t20139\tWilliamsburg\tKS\tOsage County\tH1\n66546\t20139\tWakarusa\tKS\tOsage County\tH1\n66451\t20139\tLyndon\tKS\tOsage County\tH1\n66510\t20139\tMelvern\tKS\tOsage County\tH1\n66543\t20139\tVassar\tKS\tOsage County\tH1\n66523\t20139\tOsage city\tKS\tOsage County\tH1\n66528\t20139\tQuenemo\tKS\tOsage County\tH1\n66402\t20139\tAuburn\tKS\tOsage County\tH1\n66871\t20139\tWaverly\tKS\tOsage County\tH1\n67473\t20141\tOsborne\tKS\tOsborne County\tH1\n67474\t20141\tPortis\tKS\tOsborne County\tH1\n67658\t20141\tParadise\tKS\tOsborne County\tH1\n67485\t20141\tTipton\tKS\tOsborne County\tH1\n67673\t20141\tWaldo\tKS\tOsborne County\tH1\n67649\t20141\tLuray\tKS\tOsborne County\tH1\n67651\t20141\tNatoma\tKS\tOsborne County\tH1\n67675\t20141\tWoodston\tKS\tOsborne County\tH1\n67648\t20141\tLucas\tKS\tOsborne County\tH1\n67623\t20141\tAlton\tKS\tOsborne County\tH1\n67437\t20141\tDowns\tKS\tOsborne County\tH1\n66901\t20143\tConcordia\tKS\tOttawa County\tH1\n67455\t20143\tLincoln\tKS\tOttawa County\tH1\n67466\t20143\tMiltonvale\tKS\tOttawa County\tH1\n67470\t20143\tNew cambria\tKS\tOttawa County\tH1\n67401\t20143\tSalina\tKS\tOttawa County\tH1\n67480\t20143\tSolomon\tKS\tOttawa County\tH1\n67467\t20143\tMinneapolis\tKS\tOttawa County\tH1\n67458\t20143\tLongford\tKS\tOttawa County\tH1\n67436\t20143\tDelphos\tKS\tOttawa County\tH1\n67422\t20143\tBennington\tKS\tOttawa County\tH1\n67445\t20143\tGlasco\tKS\tOttawa County\tH1\n67432\t20143\tClay center\tKS\tOttawa County\tH1\n67484\t20143\tTescott\tKS\tOttawa County\tH1\n67418\t20143\tBarnard\tKS\tOttawa County\tH1\n67575\t20145\tRush center\tKS\tPawnee County\tH1\n67574\t20145\tRozel\tKS\tPawnee County\tH1\n67550\t20145\tLarned\tKS\tPawnee County\tH1\n67529\t20145\tGarfield\tKS\tPawnee County\tH1\n67547\t20145\tKinsley\tKS\tPawnee County\tH1\n67523\t20145\tBurdett\tKS\tPawnee County\tH1\n67557\t20145\tMacksville\tKS\tPawnee County\tH1\n67567\t20145\tPawnee rock\tKS\tPawnee County\tH1\n67644\t20147\tKirwin\tKS\tPhillips County\tH1\n67661\t20147\tPhillipsburg\tKS\tPhillips County\tH1\n67646\t20147\tLogan\tKS\tPhillips County\tH1\n67647\t20147\tLong island\tKS\tPhillips County\tH1\n67621\t20147\tAgra\tKS\tPhillips County\tH1\n66951\t20147\tKensington\tKS\tPhillips County\tH1\n67628\t20147\tCedar\tKS\tPhillips County\tH1\n67639\t20147\tGlade\tKS\tPhillips County\tH1\n67664\t20147\tPrairie view\tKS\tPhillips County\tH1\n66547\t20149\tWamego\tKS\tPottawatomie County\tH1\n66549\t20149\tWestmoreland\tKS\tPottawatomie County\tH1\n66502\t20149\tManhattan\tKS\tPottawatomie County\tH1\n66521\t20149\tOnaga\tKS\tPottawatomie County\tH1\n66536\t20149\tSaint marys\tKS\tPottawatomie County\tH1\n66535\t20149\tSaint george\tKS\tPottawatomie County\tH1\n66407\t20149\tBelvue\tKS\tPottawatomie County\tH1\n66520\t20149\tOlsburg\tKS\tPottawatomie County\tH1\n66422\t20149\tEmmett\tKS\tPottawatomie County\tH1\n66432\t20149\tHavensville\tKS\tPottawatomie County\tH1\n66540\t20149\tSoldier\tKS\tPottawatomie County\tH1\n66427\t20149\tFrankfort\tKS\tPottawatomie County\tH1\n67035\t20151\tCunningham\tKS\tPratt County\tH1\n67134\t20151\tSawyer\tKS\tPratt County\tH1\n67028\t20151\tCoats\tKS\tPratt County\tH1\n67066\t20151\tIuka\tKS\tPratt County\tH1\n67576\t20151\tSt john\tKS\tPratt County\tH1\n67021\t20151\tByers\tKS\tPratt County\tH1\n67059\t20151\tHaviland\tKS\tPratt County\tH1\n67124\t20151\tPratt\tKS\tPratt County\tH1\n67065\t20151\tIsabel\tKS\tPratt County\tH1\n67557\t20151\tMacksville\tKS\tPratt County\tH1\n67583\t20151\tTuron\tKS\tPratt County\tH1\n67749\t20153\tOberlin\tKS\tRawlins County\tH1\n67744\t20153\tLudell\tKS\tRawlins County\tH1\n67739\t20153\tHerndon\tKS\tRawlins County\tH1\n67730\t20153\tAtwood\tKS\tRawlins County\tH1\n67701\t20153\tColby\tKS\tRawlins County\tH1\n67745\t20153\tMc donald\tKS\tRawlins County\tH1\n67025\t20155\tCheney\tKS\tReno County\tH1\n67035\t20155\tCunningham\tKS\tReno County\tH1\n67501\t20155\tHutchinson\tKS\tReno County\tH1\n67522\t20155\tBuhler\tKS\tReno County\tH1\n67020\t20155\tBurrton\tKS\tReno County\tH1\n67579\t20155\tSterling\tKS\tReno County\tH1\n67514\t20155\tArlington\tKS\tReno County\tH1\n67546\t20155\tInman\tKS\tReno County\tH1\n67068\t20155\tKingman\tKS\tReno County\tH1\n67505\t20155\tSouth hutchinson\tKS\tReno County\tH1\n67543\t20155\tHaven\tKS\tReno County\tH1\n67585\t20155\tYoder\tKS\tReno County\tH1\n67578\t20155\tStafford\tKS\tReno County\tH1\n67568\t20155\tPlevna\tKS\tReno County\tH1\n67502\t20155\tHutchinson\tKS\tReno County\tH1\n67561\t20155\tNickerson\tKS\tReno County\tH1\n67512\t20155\tAlden\tKS\tReno County\tH1\n67570\t20155\tPretty prairie\tKS\tReno County\tH1\n67510\t20155\tAbbyville\tKS\tReno County\tH1\n67108\t20155\tMount hope\tKS\tReno County\tH1\n67566\t20155\tPartridge\tKS\tReno County\tH1\n67581\t20155\tSylvia\tKS\tReno County\tH1\n67583\t20155\tTuron\tKS\tReno County\tH1\n66935\t20157\tBelleville\tKS\tRepublic County\tH1\n66939\t20157\tCourtland\tKS\tRepublic County\tH1\n66901\t20157\tConcordia\tKS\tRepublic County\tH1\n66966\t20157\tScandia\tKS\tRepublic County\tH1\n66940\t20157\tCuba\tKS\tRepublic County\tH1\n66964\t20157\tRepublic\tKS\tRepublic County\tH1\n66960\t20157\tNarka\tKS\tRepublic County\tH1\n66930\t20157\tAgenda\tKS\tRepublic County\tH1\n66959\t20157\tMunden\tKS\tRepublic County\tH1\n66949\t20157\tJewell\tKS\tRepublic County\tH1\n66948\t20157\tJamestown\tKS\tRepublic County\tH1\n66961\t20157\tNorway\tKS\tRepublic County\tH1\n66938\t20157\tClyde\tKS\tRepublic County\tH1\n67573\t20159\tRaymond\tKS\tRice County\tH1\n67459\t20159\tLorraine\tKS\tRice County\tH1\n67579\t20159\tSterling\tKS\tRice County\tH1\n67546\t20159\tInman\tKS\tRice County\tH1\n67524\t20159\tChase\tKS\tRice County\tH1\n67526\t20159\tEllinwood\tKS\tRice County\tH1\n67502\t20159\tHutchinson\tKS\tRice County\tH1\n67444\t20159\tGeneseo\tKS\tRice County\tH1\n67457\t20159\tLittle river\tKS\tRice County\tH1\n67561\t20159\tNickerson\tKS\tRice County\tH1\n67427\t20159\tBushton\tKS\tRice County\tH1\n67512\t20159\tAlden\tKS\tRice County\tH1\n67491\t20159\tWindom\tKS\tRice County\tH1\n67554\t20159\tLyons\tKS\tRice County\tH1\n66442\t20161\tFort riley\tKS\tRiley County\tH1\n66554\t20161\tRandolph\tKS\tRiley County\tH1\n66531\t20161\tRiley\tKS\tRiley County\tH1\n66933\t20161\tBarnes\tKS\tRiley County\tH1\n67447\t20161\tGreen\tKS\tRiley County\tH1\n66505\t20161\tManhattan\tKS\tRiley County\tH1\n66502\t20161\tManhattan\tKS\tRiley County\tH1\n66548\t20161\tWaterville\tKS\tRiley County\tH1\n66517\t20161\tOgden\tKS\tRiley County\tH1\n66449\t20161\tLeonardville\tKS\tRiley County\tH1\n66411\t20161\tBlue rapids\tKS\tRiley County\tH1\n66503\t20161\tManhattan\tKS\tRiley County\tH1\n66514\t20161\tMilford\tKS\tRiley County\tH1\n66506\t20161\tManhattan\tKS\tRiley County\tH1\n67432\t20161\tClay center\tKS\tRiley County\tH1\n67659\t20163\tPenokee\tKS\tRooks County\tH1\n67651\t20163\tNatoma\tKS\tRooks County\tH1\n67661\t20163\tPhillipsburg\tKS\tRooks County\tH1\n67663\t20163\tPlainville\tKS\tRooks County\tH1\n67669\t20163\tStockton\tKS\tRooks County\tH1\n67642\t20163\tHill city\tKS\tRooks County\tH1\n67675\t20163\tWoodston\tKS\tRooks County\tH1\n67646\t20163\tLogan\tKS\tRooks County\tH1\n67632\t20163\tDamar\tKS\tRooks County\tH1\n67657\t20163\tPalco\tKS\tRooks County\tH1\n67639\t20163\tGlade\tKS\tRooks County\tH1\n67575\t20165\tRush center\tKS\tRush County\tH1\n67511\t20165\tAlbert\tKS\tRush County\tH1\n67553\t20165\tLiebenthal\tKS\tRush County\tH1\n67513\t20165\tAlexander\tKS\tRush County\tH1\n67548\t20165\tLa crosse\tKS\tRush County\tH1\n67565\t20165\tOtis\tKS\tRush County\tH1\n67559\t20165\tNekoma\tKS\tRush County\tH1\n67521\t20165\tBrownell\tKS\tRush County\tH1\n67567\t20165\tPawnee rock\tKS\tRush County\tH1\n67556\t20165\tMc cracken\tKS\tRush County\tH1\n67520\t20165\tBison\tKS\tRush County\tH1\n67665\t20167\tRussell\tKS\tRussell County\tH1\n67658\t20167\tParadise\tKS\tRussell County\tH1\n67673\t20167\tWaldo\tKS\tRussell County\tH1\n67649\t20167\tLuray\tKS\tRussell County\tH1\n67640\t20167\tGorham\tKS\tRussell County\tH1\n67490\t20167\tWilson\tKS\tRussell County\tH1\n67648\t20167\tLucas\tKS\tRussell County\tH1\n67626\t20167\tBunker hill\tKS\tRussell County\tH1\n67634\t20167\tDorrance\tKS\tRussell County\tH1\n67544\t20167\tHoisington\tKS\tRussell County\tH1\n67481\t20167\tSylvan grove\tKS\tRussell County\tH1\n67448\t20169\tGypsum\tKS\tSaline County\tH1\n67402\t20169\tSalina\tKS\tSaline County\tH1\n67470\t20169\tNew cambria\tKS\tSaline County\tH1\n67401\t20169\tSalina\tKS\tSaline County\tH1\n67416\t20169\tAssaria\tKS\tSaline County\tH1\n67480\t20169\tSolomon\tKS\tSaline County\tH1\n67425\t20169\tBrookville\tKS\tSaline County\tH1\n67456\t20169\tLindsborg\tKS\tSaline County\tH1\n67464\t20169\tMarquette\tKS\tSaline County\tH1\n67484\t20169\tTescott\tKS\tSaline County\tH1\n67442\t20169\tFalun\tKS\tSaline County\tH1\n67851\t20171\tHolcomb\tKS\tScott County\tH1\n67863\t20171\tMarienthal\tKS\tScott County\tH1\n67850\t20171\tHealy\tKS\tScott County\tH1\n67871\t20171\tScott city\tKS\tScott County\tH1\n67025\t20173\tCheney\tKS\tSedgwick County\tH1\n67026\t20173\tClearwater\tKS\tSedgwick County\tH1\n67030\t20173\tColwich\tKS\tSedgwick County\tH1\n67060\t20173\tHaysville\tKS\tSedgwick County\tH1\n67110\t20173\tMulvane\tKS\tSedgwick County\tH1\n67216\t20173\tWichita\tKS\tSedgwick County\tH1\n67020\t20173\tBurrton\tKS\tSedgwick County\tH1\n67207\t20173\tWichita\tKS\tSedgwick County\tH1\n67220\t20173\tWichita\tKS\tSedgwick County\tH1\n67210\t20173\tWichita\tKS\tSedgwick County\tH1\n67232\t20173\tWichita\tKS\tSedgwick County\tH1\n67260\t20173\tWichita\tKS\tSedgwick County\tH1\n67050\t20173\tGarden plain\tKS\tSedgwick County\tH1\n67205\t20173\tWichita\tKS\tSedgwick County\tH1\n67226\t20173\tWichita\tKS\tSedgwick County\tH1\n67230\t20173\tWichita\tKS\tSedgwick County\tH1\n67204\t20173\tWichita\tKS\tSedgwick County\tH1\n67201\t20173\tWichita\tKS\tSedgwick County\tH1\n67135\t20173\tSedgwick\tKS\tSedgwick County\tH1\n67147\t20173\tValley center\tKS\tSedgwick County\tH1\n67543\t20173\tHaven\tKS\tSedgwick County\tH1\n67055\t20173\tGreenwich\tKS\tSedgwick County\tH1\n67275\t20173\tWichita\tKS\tSedgwick County\tH1\n67031\t20173\tConway springs\tKS\tSedgwick County\tH1\n67218\t20173\tWichita\tKS\tSedgwick County\tH1\n67214\t20173\tWichita\tKS\tSedgwick County\tH1\n67221\t20173\tMcconnell afb\tKS\tSedgwick County\tH1\n67277\t20173\tWichita\tKS\tSedgwick County\tH1\n67223\t20173\tWichita\tKS\tSedgwick County\tH1\n67227\t20173\tWichita\tKS\tSedgwick County\tH1\n67149\t20173\tViola\tKS\tSedgwick County\tH1\n67039\t20173\tDouglass\tKS\tSedgwick County\tH1\n67017\t20173\tBenton\tKS\tSedgwick County\tH1\n67052\t20173\tGoddard\tKS\tSedgwick County\tH1\n67213\t20173\tWichita\tKS\tSedgwick County\tH1\n67133\t20173\tRose hill\tKS\tSedgwick County\tH1\n67228\t20173\tWichita\tKS\tSedgwick County\tH1\n67235\t20173\tWichita\tKS\tSedgwick County\tH1\n67001\t20173\tAndale\tKS\tSedgwick County\tH1\n67202\t20173\tWichita\tKS\tSedgwick County\tH1\n67215\t20173\tWichita\tKS\tSedgwick County\tH1\n67067\t20173\tKechi\tKS\tSedgwick County\tH1\n67276\t20173\tWichita\tKS\tSedgwick County\tH1\n67120\t20173\tPeck\tKS\tSedgwick County\tH1\n67212\t20173\tWichita\tKS\tSedgwick County\tH1\n67203\t20173\tWichita\tKS\tSedgwick County\tH1\n67208\t20173\tWichita\tKS\tSedgwick County\tH1\n67209\t20173\tWichita\tKS\tSedgwick County\tH1\n67217\t20173\tWichita\tKS\tSedgwick County\tH1\n67219\t20173\tWichita\tKS\tSedgwick County\tH1\n67106\t20173\tMilton\tKS\tSedgwick County\tH1\n67037\t20173\tDerby\tKS\tSedgwick County\tH1\n67016\t20173\tBentley\tKS\tSedgwick County\tH1\n67108\t20173\tMount hope\tKS\tSedgwick County\tH1\n67211\t20173\tWichita\tKS\tSedgwick County\tH1\n67206\t20173\tWichita\tKS\tSedgwick County\tH1\n67101\t20173\tMaize\tKS\tSedgwick County\tH1\n67118\t20173\tNorwich\tKS\tSedgwick County\tH1\n67278\t20173\tWichita\tKS\tSedgwick County\tH1\n67951\t20175\tHugoton\tKS\tSeward County\tH1\n67954\t20175\tRolla\tKS\tSeward County\tH1\n67869\t20175\tPlains\tKS\tSeward County\tH1\n67870\t20175\tSatanta\tKS\tSeward County\tH1\n67877\t20175\tSublette\tKS\tSeward County\tH1\n67859\t20175\tKismet\tKS\tSeward County\tH1\n67901\t20175\tLiberal\tKS\tSeward County\tH1\n67952\t20175\tMoscow\tKS\tSeward County\tH1\n66414\t20177\tCarbondale\tKS\tShawnee County\tH1\n66431\t20177\tHarveyville\tKS\tShawnee County\tH1\n66611\t20177\tTopeka\tKS\tShawnee County\tH1\n66605\t20177\tTopeka\tKS\tShawnee County\tH1\n66610\t20177\tTopeka\tKS\tShawnee County\tH1\n66630\t20177\tTopeka\tKS\tShawnee County\tH1\n66539\t20177\tSilver lake\tKS\tShawnee County\tH1\n66617\t20177\tTopeka\tKS\tShawnee County\tH1\n66050\t20177\tLecompton\tKS\tShawnee County\tH1\n66512\t20177\tMeriden\tKS\tShawnee County\tH1\n66619\t20177\tTopeka\tKS\tShawnee County\tH1\n66601\t20177\tTopeka\tKS\tShawnee County\t
